vi "Testbench for 1C.1 Camera - PixelToUTM and UTMToPixel.vi"() -> ()   [LabVIEW 2011]
uses:
  2-Think/2 Typedefs/UTM Location.ctl
panel:
  out "Converted back to UTM location":T1
  out "Converted to pixel location":cluster{"X":i32, "Y":i32}
  in  "UTM Location":T1
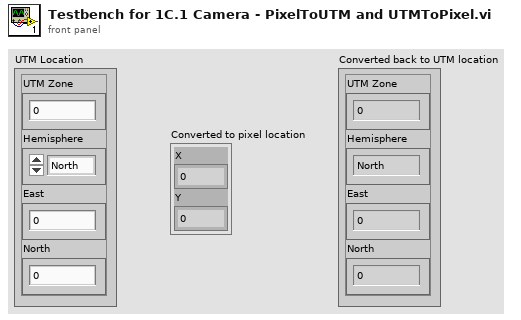
[diagram p1: front panel]
types:
  T1 = typedef "UTM Location.ctl" = cluster{"UTM Zone":dbl, "Hemisphere":enum16{"North", "South"}, "East":dbl, "North":dbl}
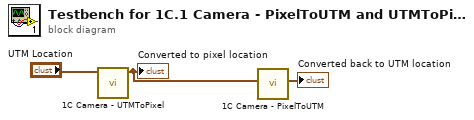
[diagram p0: block diagram]
diagram:
  n1 = call "1C Camera - UTMToPixel.vi"("Robot UTM Location in"="UTM Location") -> ("output pixels cluster"=w3:cluster{"X":i32, "Y":i32})  [unwired: 10 in]
  "Converted to pixel location" <- w3
  n2 = call "1C Camera - PixelToUTM.vi"("Found Marker Position in (pixels)"=w3) -> ("UTM Location Out"=→"Converted back to UTM location":T1)  [unwired: 10 in]
